vi "UI.vi"(0 "Add.lvclass":refnum<class "Add.lvclass">, 5 "Num 1":dbl, 7 "Num 2":dbl, 11 "Error In":errorcluster) -> (4 "Add.lvclass 2":refnum<class "Add.lvclass">, 6 "Output":dbl, 15 "error out":errorcluster)   [LabVIEW 2020, in "Add.lvclass"]
uses:
  Add.lvclass
  D:/Github Projects/LV_Assignment/Tasks/A17/Calculator_using_instance/Classes/Arithmetic_Operations/Arithmetic_Operations.lvclass
  Typedef's/UserEvent_Operations.ctl
  Add.lvclass/Add.ctl
  Arithmetic_Operations/Arithmetic_Operations.lvclass
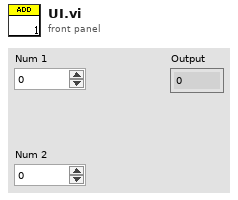
[diagram p1: front panel]
types:
  T1 = typedef "UserEvent_Operations.ctl" = enum16{"Create", "Generate", "Get Ref", "Destroy"}
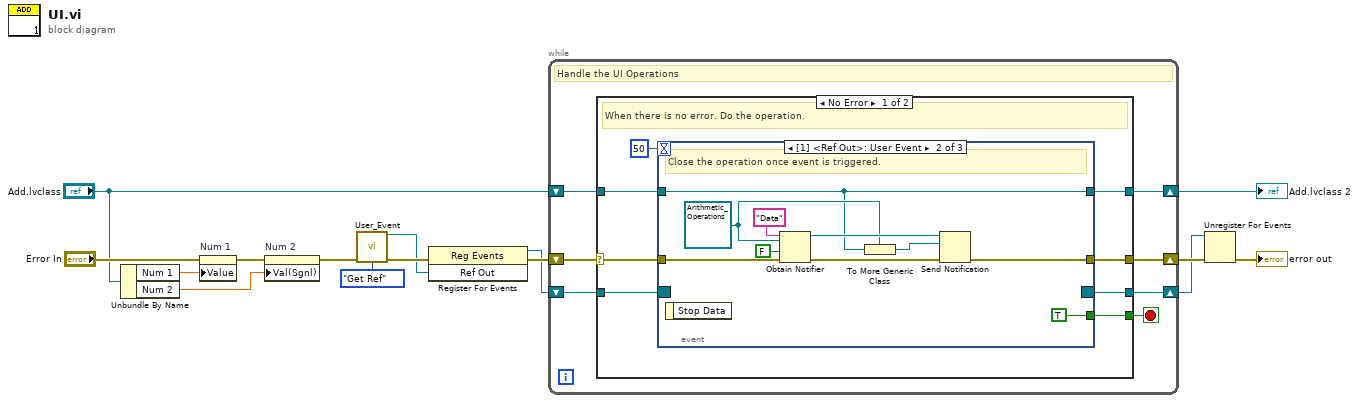
[diagram p0: block diagram]
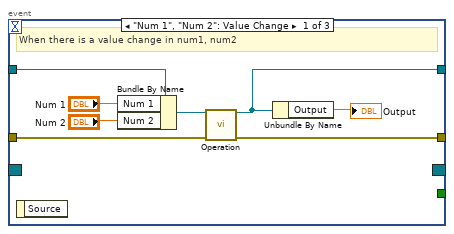
[diagram p2: hidden frame]
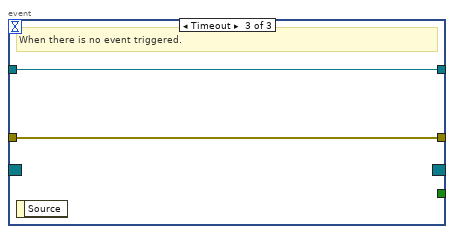
[diagram p3: hidden frame]
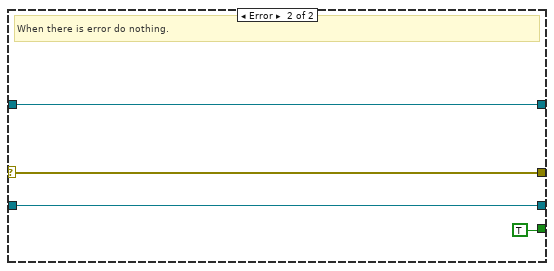
[diagram p4: hidden frame]
diagram:
  n1 = Unbundle By Name("Add.lvclass") -> ("Num 1"=w9:dbl, "Num 2"=w8:dbl)
  n2 = property on="Num 1" class="DigNum (strict)"(error in="Error In", "Value"=w9) -> (error out=w12:errorcluster)  [unwired: 1 in, 1 out]
  n3 = property on="Num 2" class="DigNum (strict)"(error in=w12, "Val(Sgnl)"=w8) -> (error out=w11:errorcluster)  [unwired: 1 in, 1 out]
  n4 = call "User_Event.vi"("Error In"=w11, "Enum"=UserEvent_Operations."Get Ref") -> ("Ref Out"=w4:refnum<user-event>, "Error Out"=w7:errorcluster)  [unwired: 12 in]
  n5 = register-events(error in=w7, w4) -> (reference out=w3:refnum<event-registration>, error out=w5:errorcluster)  [unwired: 1 in]
  n6 = while {
    shift-right: [w20] -> w14
    shift-left: w5 -> [w22]
    shift-right: [w19] -> w13
    shift-left: "Add.lvclass" -> [w21]
    shift-right: [w17] -> w1
    shift-left: w3 -> [w18]
    stop <- w16 stop-if-true
    # "Handle the UI Operations"
    n7 = case shown="No Error" w22 {
      selector: w22 -> [w30 w53]
      tunnel: w21 -> [w29 w54]
      tunnel: [w28 w53] -> w20
      tunnel: [w27 w54] -> w19
      tunnel: w18 -> [w25 w52]
      tunnel: [w24 w52] -> w17
      tunnel: [w23 TRUE] -> w16
      frame No Error {
        # "When there is no error. Do the operation."
        n8 = event shown="[1] <Ref Out>: User Event" {
          selector: w25 -> [_ _ _]
          dyn-events: [_ _ _] -> w24
          timeout: 50 -> [_ _ _]
          tunnel: w30 -> [w33 w48 w49]
          tunnel: w29 -> [w38 w41 w50]
          tunnel: [w34 w44 w49] -> w28
          tunnel: [w32 w41 w50] -> w27
          tunnel: [_ TRUE _] -> w23
          event "Num 1", "Num 2": Value Change {
            # "When there is a value change in num1, num2"
            n9 = event-data() -> ()  [unwired: 1 in, 1 out]
            n10 = Bundle By Name(cluster=w38, "Num 1"="Num 1", "Num 2"="Num 2") -> (w35:refnum<class "Add.lvclass">)
            n11 = call-dynamic "Operation.vi"("Add in"=w35, "Error In"=w33) -> ("Add out"=w32:refnum<class "Add.lvclass">, "Error Out"=w34:errorcluster)  [unwired: 12 in]
            n12 = Unbundle By Name(w32) -> ("Output"=→"Output":dbl)
          }
          event User Event {
            w42 = refnum<class "Arithmetic_Operations.lvclass"> refnum ("Arithmetic_Operations.lvclass")
            # "Close the operation once event is triggered."
            n13 = event-data() -> ()  [unwired: 1 in, 1 out]
            n14 = Obtain Notifier(name (unnamed)="Data", notification data type=w42, create if not found? (T)=FALSE, error in (no error)=w48) -> (notifier out=w43:refnum<notifier>, error out=w39:errorcluster)  [unwired: 1 out]
            n15 = To More Generic Class(target class=w42, reference=w41) -> (generic class reference=w40:refnum<class "Arithmetic_Operations.lvclass">)
            n16 = Send Notification(notification=w40, notifier=w43, error in (no error)=w39) -> (error out=w44:errorcluster)  [unwired: 1 out]
          }
          event Timeout {
            # "When there is no event triggered."
            n17 = event-data() -> ()  [unwired: 1 in, 1 out]
          }
        }
      }
      frame Error {
        # "When there is error do nothing."
      }
    }
  }
  "Add.lvclass 2" <- w13
  n18 = Unregister For Events(event registration refnum=w1, error in=w14) -> (error out=→"error out":errorcluster)
